vi "Read Text File.vi"(8 "error in (no error)":errorcluster, 11 "Path":path) -> (0 "error out":errorcluster, 3 "Data":dbl[](array[numeric]))   [LabVIEW 2020]
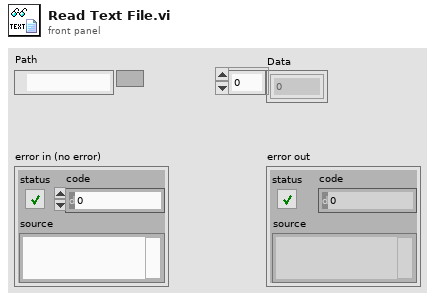
[diagram p1: front panel]
types:
  T1 = enum16{"open", "replace", "create", "open or create", "replace or create", "replace or create with confirmation"}
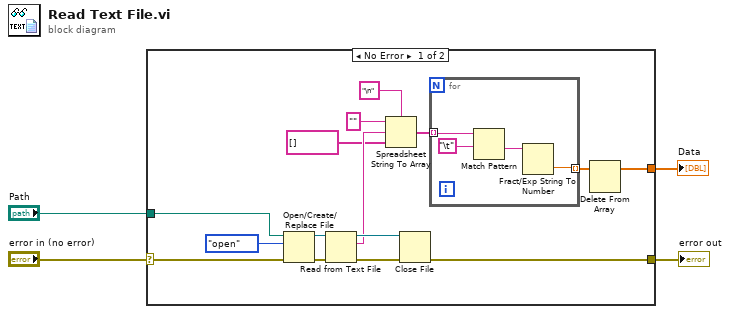
[diagram p0: block diagram]
diagram:
  n1 = case shown="No Error" "error in (no error)" {
    selector: "error in (no error)" -> [w19 w24]
    tunnel: [w17 w24] -> w3
    tunnel: "Path" -> [w18 _]
    tunnel: [w5 _] -> w1
    frame No Error {
      n2 = Open/Create/Replace File(file path (use dialog)=w18, error in=w19, operation (0:open)=T1."open") -> (refnum out=w14:refnum<file>, error out=w15:errorcluster)  [unwired: 3 in, 1 out]
      n3 = Read from Text File(file (use dialog)=w14, error in=w15) -> (refnum out=w13:refnum<file>, text=w11:string, error out=w12:errorcluster)  [unwired: 2 in, 1 out]
      n4 = Spreadsheet String To Array(delimiter (Tab)="\n", format string="", spreadsheet string=w11, array type (2D Dbl)=string[] []) -> (array=w7:string[])
      n5 = Close File(refnum=w13, error in=w12) -> (error out=w17:errorcluster)  [unwired: 1 out]
      n6 = for {
        tunnel: w7 -> [w23] mode=indexing
        tunnel: [w20] -> w6 mode=indexing
        n7 = Match Pattern(string=w23, regular expression="\t") -> (after substring=w21:string)  [unwired: 1 in, 3 out]
        n8 = Fract/Exp String To Number(string=w21) -> (number=w20:dbl)  [unwired: 3 in, 1 out]
      }
      n9 = Delete From Array(array=w6) -> (array with subset deleted=w5:dbl[])  [unwired: 2 in, 1 out]
    }
    frame Error {
    }
  }
  "error out" <- w3
  "Data" <- w1
